vi "deleave_bitpacking.vi"(11 "Data":u64[](array[numeric])) -> (2 "Counts":i16[][](array[numeric]), 3 "Voltage":dbl[][](array[numeric]))   [LabVIEW 2014]
doc: "Deleave and convert Data. Deleaves data from DMA readout and converts with SubVIs to counts and voltages."
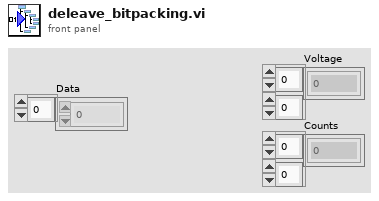
[diagram p1: front panel]
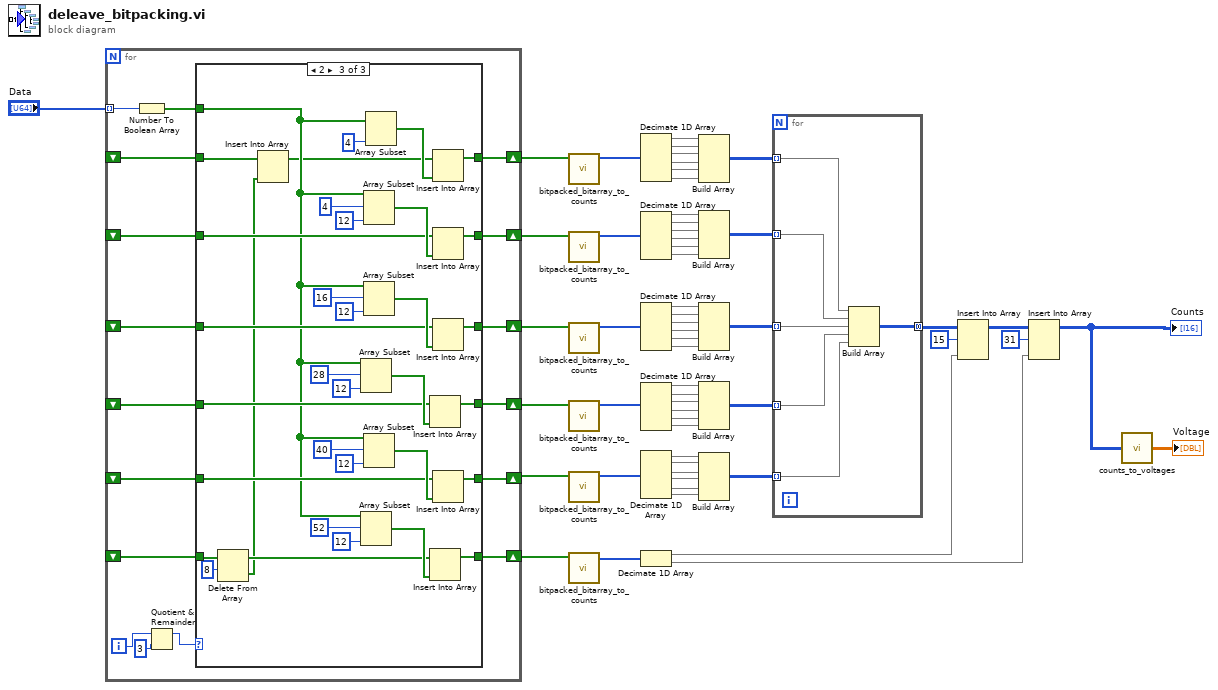
[diagram p0: block diagram]
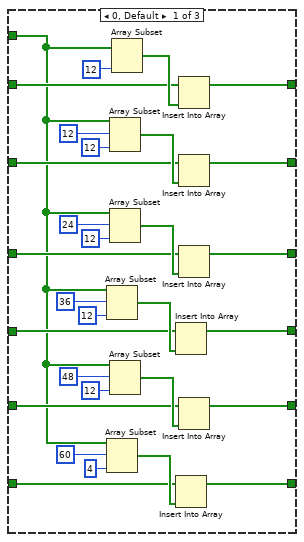
[diagram p2: hidden frame]
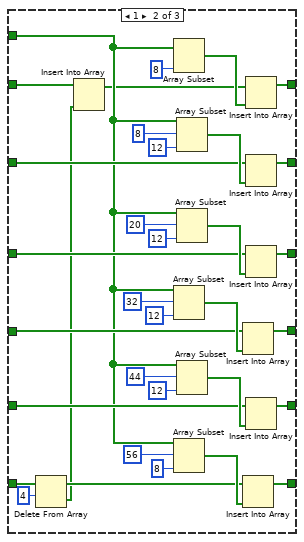
[diagram p3: hidden frame]
diagram:
  n1 = for {
    tunnel: "Data" -> [w70] mode=indexing
    shift-right: [w68] -> w55
    shift-left: _ -> [w67]
    shift-right: [w65] -> w54
    shift-left: _ -> [w66]
    shift-right: [w64] -> w53
    shift-left: _ -> [w63]
    shift-right: [w62] -> w52
    shift-left: _ -> [w61]
    shift-right: [w60] -> w51
    shift-left: _ -> [w59]
    shift-right: [w58] -> w50
    shift-left: _ -> [w57]
    i -> [w73]
    n2 = Number To Boolean Array(number=w70) -> (Boolean array=w69:bool[])
    n3 = Quotient & Remainder(x=w73, y=3) -> (x-y*floor(x/y)=w71:i32)  [unwired: 1 out]
    n4 = case shown="2" w71 {
      tunnel: w69 -> [w76 w111 w144]
      tunnel: [w99 w133 w167] -> w68
      tunnel: w67 -> [w97 w106 w140]
      tunnel: w66 -> [w96 w131 w165]
      tunnel: [w95 w130 w164] -> w65
      tunnel: [w91 w126 w160] -> w64
      tunnel: w63 -> [w90 w125 w159]
      tunnel: [w86 w121 w155] -> w62
      tunnel: w61 -> [w85 w120 w154]
      tunnel: [w81 w116 w150] -> w60
      tunnel: w59 -> [w80 w115 w149]
      tunnel: [w75 w110 w145] -> w58
      tunnel: w57 -> [w74 w109 w143]
      frame 0, Default {
        n5 = Array Subset(array=w76, index=36, length=12 ("index")) -> (w87:bool[])
        n6 = Array Subset(array=w76, index=60, length=4 ("index")) -> (w77:bool[])
        n7 = Array Subset(array=w76, index=12, length=12 ("index")) -> (w98:bool[])
        n8 = Array Subset(array=w76, index=24, length=12 ("index")) -> (w92:bool[])
        n9 = Array Subset(array=w76, index=48, length=12 ("index")) -> (w82:bool[])
        n10 = Array Subset(array=w76, length=12 ("index")) -> (w100:bool[])  [unwired: 1 in]
        n11 = Insert Into Array(array=w85, new element=w87) -> (w86:bool[])  [unwired: 1 in]
        n12 = Insert Into Array(array=w74, new element=w77) -> (w75:bool[])  [unwired: 1 in]
        n13 = Insert Into Array(array=w97, new element=w100) -> (w99:bool[])  [unwired: 1 in]
        n14 = Insert Into Array(array=w96, new element=w98) -> (w95:bool[])  [unwired: 1 in]
        n15 = Insert Into Array(array=w90, new element=w92) -> (w91:bool[])  [unwired: 1 in]
        n16 = Insert Into Array(array=w80, new element=w82) -> (w81:bool[])  [unwired: 1 in]
      }
      frame 1 {
        n17 = Delete From Array(array=w109, length=4) -> (deleted portion=w104:bool[], array with subset deleted=w108:bool[])  [unwired: 1 in]
        n18 = Insert Into Array(array=w106, new element=w104) -> (w105:bool[])  [unwired: 1 in]
        n19 = Array Subset(array=w111, length=8 ("index")) -> (w134:bool[])  [unwired: 1 in]
        n20 = Array Subset(array=w111, index=32, length=12 ("index")) -> (w122:bool[])
        n21 = Array Subset(array=w111, index=56, length=8 ("index")) -> (w112:bool[])
        n22 = Array Subset(array=w111, index=8, length=12 ("index")) -> (w132:bool[])
        n23 = Array Subset(array=w111, index=20, length=12 ("index")) -> (w127:bool[])
        n24 = Array Subset(array=w111, index=44, length=12 ("index")) -> (w117:bool[])
        n25 = Insert Into Array(array=w120, new element=w122) -> (w121:bool[])  [unwired: 1 in]
        n26 = Insert Into Array(array=w108, new element=w112) -> (w110:bool[])  [unwired: 1 in]
        n27 = Insert Into Array(array=w105, new element=w134) -> (w133:bool[])  [unwired: 1 in]
        n28 = Insert Into Array(array=w131, new element=w132) -> (w130:bool[])  [unwired: 1 in]
        n29 = Insert Into Array(array=w125, new element=w127) -> (w126:bool[])  [unwired: 1 in]
        n30 = Insert Into Array(array=w115, new element=w117) -> (w116:bool[])  [unwired: 1 in]
      }
      frame 2 {
        n31 = Delete From Array(array=w143, length=8) -> (deleted portion=w138:bool[], array with subset deleted=w142:bool[])  [unwired: 1 in]
        n32 = Insert Into Array(array=w140, new element=w138) -> (w139:bool[])  [unwired: 1 in]
        n33 = Array Subset(array=w144, index=28, length=12 ("index")) -> (w156:bool[])
        n34 = Array Subset(array=w144, index=52, length=12 ("index")) -> (w146:bool[])
        n35 = Array Subset(array=w144, index=4, length=12 ("index")) -> (w166:bool[])
        n36 = Array Subset(array=w144, index=16, length=12 ("index")) -> (w161:bool[])
        n37 = Array Subset(array=w144, index=40, length=12 ("index")) -> (w151:bool[])
        n38 = Array Subset(array=w144, length=4 ("index")) -> (w168:bool[])  [unwired: 1 in]
        n39 = Insert Into Array(array=w154, new element=w156) -> (w155:bool[])  [unwired: 1 in]
        n40 = Insert Into Array(array=w142, new element=w146) -> (w145:bool[])  [unwired: 1 in]
        n41 = Insert Into Array(array=w139, new element=w168) -> (w167:bool[])  [unwired: 1 in]
        n42 = Insert Into Array(array=w165, new element=w166) -> (w164:bool[])  [unwired: 1 in]
        n43 = Insert Into Array(array=w159, new element=w161) -> (w160:bool[])  [unwired: 1 in]
        n44 = Insert Into Array(array=w149, new element=w151) -> (w150:bool[])  [unwired: 1 in]
      }
    }
  }
  n45 = call "bitpacked_bitarray_to_counts.vi"("Bit Array"=w55) -> ("Integer Array"=w49:i16[])  [unwired: 10 in]
  n46 = call "bitpacked_bitarray_to_counts.vi"("Bit Array"=w54) -> ("Integer Array"=w48:i16[])  [unwired: 10 in]
  n47 = call "bitpacked_bitarray_to_counts.vi"("Bit Array"=w53) -> ("Integer Array"=w47:i16[])  [unwired: 10 in]
  n48 = call "bitpacked_bitarray_to_counts.vi"("Bit Array"=w52) -> ("Integer Array"=w46:i16[])  [unwired: 10 in]
  n49 = call "bitpacked_bitarray_to_counts.vi"("Bit Array"=w51) -> ("Integer Array"=w45:i16[])  [unwired: 10 in]
  n50 = call "bitpacked_bitarray_to_counts.vi"("Bit Array"=w50) -> ("Integer Array"=w44:i16[])  [unwired: 10 in]
  n51 = Decimate 1D Array(w49) -> (w43:i16[], w42:i16[], w41:i16[], w40:i16[], w39:i16[], w38:i16[])
  n52 = Decimate 1D Array(w48) -> (w37:i16[], w36:i16[], w35:i16[], w34:i16[], w33:i16[], w32:i16[])
  n53 = Decimate 1D Array(w47) -> (w31:i16[], w30:i16[], w29:i16[], w28:i16[], w27:i16[], w26:i16[])
  n54 = Decimate 1D Array(w46) -> (w25:i16[], w24:i16[], w23:i16[], w22:i16[], w21:i16[], w20:i16[])
  n55 = Decimate 1D Array(w45) -> (w19:i16[], w18:i16[], w17:i16[], w16:i16[], w15:i16[], w14:i16[])
  n56 = Decimate 1D Array(w44) -> (w6:i16[], w3:i16[])
  n57 = Build Array(w43, w42, w41, w40, w39, w38) -> (w13:i16[][])
  n58 = Build Array(w37, w36, w35, w34, w33, w32) -> (w12:i16[][])
  n59 = Build Array(w31, w30, w29, w28, w27, w26) -> (w11:i16[][])
  n60 = Build Array(w25, w24, w23, w22, w21, w20) -> (w10:i16[][])
  n61 = Build Array(w19, w18, w17, w16, w15, w14) -> (w9:i16[][])
  n62 = for {
    tunnel: w13 -> [w177] mode=indexing
    tunnel: w12 -> [w176] mode=indexing
    tunnel: w11 -> [w175] mode=indexing
    tunnel: w10 -> [w174] mode=indexing
    tunnel: w9 -> [w173] mode=indexing
    tunnel: [w172] -> w8 mode=concatenating
    n63 = Build Array(w177, w176, w175, w174, w173) -> (w172:i16[][])
  }
  n64 = Insert Into Array(array=w8, index (row)=15, new element=w6) -> (w5:i16[][])  [unwired: 1 in]
  n65 = Insert Into Array(array=w5, index (row)=31, new element=w3) -> (w1:i16[][])  [unwired: 1 in]
  "Counts" <- w1
  n66 = call "counts_to_voltages.vi"("Count Array"=w1) -> ("Voltage Array"=→"Voltage":dbl[][])
